vi "Main.vi"(8 "error in":errorcluster, 11 "gRPC Server in":refnum<class "gRPC Server.lvclass">) -> (0 "error out":errorcluster, 3 "gRPC Server out":refnum<class "gRPC Server.lvclass">)   [LabVIEW 2019, in "gRPC Server (template.proto).lvlib" / "gRPC Server.lvclass"]
doc: "The <b>Queued Message Handler</b> of the Worker that owns this VI."
uses:
  gRPC Server.lvclass
  C:/Program Files (x86)/National Instruments/LabVIEW 2019/vi.lib/addons/_Workers/Library/Classes/Worker/Worker.lvclass
  Generated_server/RPC Service/Session/Session.lvclass
  Generated_server/RPC Service/Session/Session.lvclass/Session.ctl
  rql_New Client Connection.ctl
  <vilib>/gRPC/LabVIEW gRPC Library/Shared/grpcId.ctl
  Initialization Data.ctl
  Response Cases.ctl
  <vilib>/addons/_Workers/Library/Case Label.ctl
  gRPC Server.lvclass/gRPC Server.ctl
  rsp_Connection Notify.ctl
  gRPC Read/Initialization Data.ctl
  gRPC Read/Response Cases.ctl
  rwr_Create gRPC Server.ctl
  rwr_Create gRPC Server Reply.ctl
  rwr_Destroy gRPC Server.ctl
  rwr_Destroy gRPC Server Reply.ctl
  rqp_Msg_ToClient_1.ctl
  Generated_server/RPC Messages/w4lvgrpc_Msg_ToClient_1.ctl
  Generated_server/RPC Messages/w4lvgrpc_ToClient.ctl
  Generated_server/RPC Messages/w4lvgrpc_ToClient_payload/w4lvgrpc_ToClient_payload.lvclass
  Generated_server/RPC Messages/w4lvgrpc_ToClient_payload/w4lvgrpc_ToClient_payload.lvclass/w4lvgrpc_ToClient_payload.ctl
  rqp_Msg_ToClient_2.ctl
  Generated_server/RPC Messages/w4lvgrpc_Msg_ToClient_2.ctl
  rqp_Msg_ToClient_3.ctl
  Generated_server/RPC Messages/w4lvgrpc_Msg_ToClient_3.ctl
  rqp_Msg_ToClient_4.ctl
  Generated_server/RPC Messages/w4lvgrpc_Msg_ToClient_4.ctl
  rqp_Msg_ToClient_5.ctl
  Generated_server/RPC Messages/w4lvgrpc_Msg_ToClient_5.ctl
  rqp_Msg_ToClient_6.ctl
  Generated_server/RPC Messages/w4lvgrpc_Msg_ToClient_6.ctl
  rqp_Msg_ToClient_7.ctl
  Generated_server/RPC Messages/w4lvgrpc_Msg_ToClient_7.ctl
  rqp_Msg_ToClient_8.ctl
  Generated_server/RPC Messages/w4lvgrpc_Msg_ToClient_8.ctl
  rqp_Msg_ToClient_9.ctl
  Generated_server/RPC Messages/w4lvgrpc_Msg_ToClient_9.ctl
  Generated_server/RPC Messages/w4lvgrpc_ToServer_payload/w4lvgrpc_ToServer_payload.lvclass/w4lvgrpc_ToServer_payload.ctl
  rsp_Msg_ToServer_1.ctl
  Generated_server/RPC Messages/w4lvgrpc_Msg_ToServer_1.ctl
  rsp_Msg_ToServer_2.ctl
  Generated_server/RPC Messages/w4lvgrpc_Msg_ToServer_2.ctl
  rsp_Msg_ToServer_3.ctl
  Generated_server/RPC Messages/w4lvgrpc_Msg_ToServer_3.ctl
  rsp_Msg_ToServer_4.ctl
  Generated_server/RPC Messages/w4lvgrpc_Msg_ToServer_4.ctl
  rsp_Msg_ToServer_5.ctl
  Generated_server/RPC Messages/w4lvgrpc_Msg_ToServer_5.ctl
  rsp_Msg_ToServer_6.ctl
  Generated_server/RPC Messages/w4lvgrpc_Msg_ToServer_6.ctl
  rsp_Msg_ToServer_7.ctl
  Generated_server/RPC Messages/w4lvgrpc_Msg_ToServer_7.ctl
  rsp_Msg_ToServer_8.ctl
  Generated_server/RPC Messages/w4lvgrpc_Msg_ToServer_8.ctl
  rsp_Msg_ToServer_9.ctl
  Generated_server/RPC Messages/w4lvgrpc_Msg_ToServer_9.ctl
  Generated_server/RPC Messages/Set w4lvgrpc_ToClient.vi
  Generated_server/RPC Messages/Set w4lvgrpc_ToClient.vi/dcc74a39-081a-4bdd-860b-8ed792803c96.vi
  Generated_server/RPC Messages/RichToFlatw4lvgrpc_ToClient.vi
  <vilib>/gRPC/LabVIEW gRPC Library/Shared/TranslateGrpcError.vi
  Generated_server/RPC Messages/RichToFlatw4lvgrpc_Msg_ToClient_1.vi
  Generated_server/RPC Messages/RichToFlatw4lvgrpc_Msg_ToClient_2.vi
  Generated_server/RPC Messages/RichToFlatw4lvgrpc_Msg_ToClient_3.vi
  Generated_server/RPC Messages/RichToFlatw4lvgrpc_Msg_ToClient_4.vi
  Generated_server/RPC Messages/RichToFlatw4lvgrpc_Msg_ToClient_5.vi
  Generated_server/RPC Messages/RichToFlatw4lvgrpc_Msg_ToClient_6.vi
  Generated_server/RPC Messages/RichToFlatw4lvgrpc_Msg_ToClient_7.vi
  Generated_server/RPC Messages/RichToFlatw4lvgrpc_Msg_ToClient_8.vi
  Generated_server/RPC Messages/RichToFlatw4lvgrpc_Msg_ToClient_9.vi
  <vilib>/Utility/error.llb/Error Cluster From Error Code.vi
  <vilib>/gRPC/LabVIEW gRPC Library/Server API/Server/Get Server DLL Path.vi
  <vilib>/addons/_Workers/Library/Classes/Message Queue/Message Queue.lvclass
  <vilib>/ErrorRing/Error Ring.xnode
  <vilib>/addons/_Workers/Library/Workers.lvlib
  gRPC Read/gRPC Read.lvclass
  Generated_server/RPC Messages/w4lvgrpc_ToServer_payload/w4lvgrpc_ToServer_payload.lvclass
  Generated_server/Generated_server.lvlib
  <vilib>/gRPC/LabVIEW gRPC Library/grpc-lvsupport-release.lvlib
  <vilib>/gRPC/LabVIEW gRPC Servicer/Servicer/Servicer.lvclass
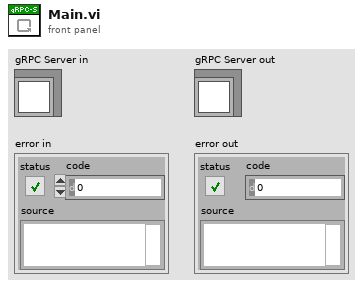
[diagram p1: front panel]
types:
  T1 = typedef "gRPC Server (template.proto).lvlib/gRPC Server.lvclass/rql_New Client Connection.ctl" = cluster{"gRPC ID":T2}
  T2 = typedef "grpc-lvsupport-release.lvlib/grpcId.ctl" = u64
  T3 = typedef "gRPC Server (template.proto).lvlib/gRPC Server.lvclass/Initialization Data.ctl" = cluster{"Response Cases":T4}
  T4 = typedef "gRPC Server (template.proto).lvlib/gRPC Server.lvclass/Response Cases.ctl" = cluster{"Connection Notify":T5, "Server Error":T5, "Msg_ToServer_1":T5, "Msg_ToServer_2":T5, "Msg_ToServer_3":T5, "Msg_ToServer_4":T5, "Msg_ToServer_5":T5, "Msg_ToServer_6":T5, "Msg_ToServer_7":T5, "Msg_ToServer_8":T5, "Msg_ToServer_9":T5}
  T5 = typedef "Workers.lvlib/Case Label.ctl" = string
  T6 = typedef "gRPC Server (template.proto).lvlib/gRPC Read.lvclass/Initialization Data.ctl" = cluster{"Response Cases":T7, "gRPC ID":T2}
  T7 = typedef "gRPC Server (template.proto).lvlib/gRPC Read.lvclass/Response Cases.ctl" = cluster{"Receive Incoming Data":T5, "Connection Lost":T5, "New Connection":T5}
  T8 = typedef "gRPC Server (template.proto).lvlib/gRPC Server.lvclass/rsp_Connection Notify.ctl" = cluster{"gRPC ID":T2, "Connected?":bool}
  T9 = typedef "gRPC Server (template.proto).lvlib/gRPC Server.lvclass/rwr_Create gRPC Server Reply.ctl" = cluster{"Listening Port":i32}
  T10 = typedef "gRPC Server (template.proto).lvlib/gRPC Server.lvclass/rwr_Create gRPC Server.ctl" = cluster{"Server Key File (.key)":path, "Server Certificate File (.crt)":path, "Server Address":string}
  T11 = typedef "gRPC Server (template.proto).lvlib/gRPC Server.lvclass/rwr_Destroy gRPC Server Reply.ctl" = cluster{"String":string}
  T12 = typedef "gRPC Server (template.proto).lvlib/gRPC Server.lvclass/rwr_Destroy gRPC Server.ctl" = cluster{"Placeholder":string}
  T13 = typedef "Generated_server.lvlib/w4lvgrpc_ToClient.ctl" = cluster{"w4lvgrpc_ToClient_payload":refnum<class "w4lvgrpc_ToClient_payload.lvclass">}
  T14 = typedef "gRPC Server (template.proto).lvlib/gRPC Server.lvclass/rqp_Msg_ToClient_1.ctl" = cluster{"w4lvgrpc_Msg_ToClient_1":T15}
  T15 = typedef "Generated_server.lvlib/w4lvgrpc_Msg_ToClient_1.ctl" = cluster{"placeholder":string}
  T16 = typedef "gRPC Server (template.proto).lvlib/gRPC Server.lvclass/rqp_Msg_ToClient_2.ctl" = cluster{"w4lvgrpc_Msg_ToClient_2":T17}
  T17 = typedef "Generated_server.lvlib/w4lvgrpc_Msg_ToClient_2.ctl" = cluster{"placeholder":string}
  T18 = typedef "gRPC Server (template.proto).lvlib/gRPC Server.lvclass/rqp_Msg_ToClient_3.ctl" = cluster{"w4lvgrpc_Msg_ToClient_3":T19}
  T19 = typedef "Generated_server.lvlib/w4lvgrpc_Msg_ToClient_3.ctl" = cluster{"placeholder":string}
  T20 = typedef "gRPC Server (template.proto).lvlib/gRPC Server.lvclass/rqp_Msg_ToClient_4.ctl" = cluster{"w4lvgrpc_Msg_ToClient_4":T21}
  T21 = typedef "Generated_server.lvlib/w4lvgrpc_Msg_ToClient_4.ctl" = cluster{"placeholder":string}
  T22 = typedef "gRPC Server (template.proto).lvlib/gRPC Server.lvclass/rqp_Msg_ToClient_5.ctl" = cluster{"w4lvgrpc_Msg_ToClient_5":T23}
  T23 = typedef "Generated_server.lvlib/w4lvgrpc_Msg_ToClient_5.ctl" = cluster{"placeholder":string}
  T24 = typedef "gRPC Server (template.proto).lvlib/gRPC Server.lvclass/rqp_Msg_ToClient_6.ctl" = cluster{"w4lvgrpc_Msg_ToClient_6":T25}
  T25 = typedef "Generated_server.lvlib/w4lvgrpc_Msg_ToClient_6.ctl" = cluster{"placeholder":string}
  T26 = typedef "gRPC Server (template.proto).lvlib/gRPC Server.lvclass/rqp_Msg_ToClient_7.ctl" = cluster{"w4lvgrpc_Msg_ToClient_7":T27}
  T27 = typedef "Generated_server.lvlib/w4lvgrpc_Msg_ToClient_7.ctl" = cluster{"placeholder":string}
  T28 = typedef "gRPC Server (template.proto).lvlib/gRPC Server.lvclass/rqp_Msg_ToClient_8.ctl" = cluster{"w4lvgrpc_Msg_ToClient_8":T29}
  T29 = typedef "Generated_server.lvlib/w4lvgrpc_Msg_ToClient_8.ctl" = cluster{"placeholder":string}
  T30 = typedef "gRPC Server (template.proto).lvlib/gRPC Server.lvclass/rqp_Msg_ToClient_9.ctl" = cluster{"w4lvgrpc_Msg_ToClient_9":T31}
  T31 = typedef "Generated_server.lvlib/w4lvgrpc_Msg_ToClient_9.ctl" = cluster{"placeholder":string}
  T32 = typedef "gRPC Server (template.proto).lvlib/gRPC Server.lvclass/rsp_Msg_ToServer_1.ctl" = cluster{"w4lvgrpc_Msg_ToServer_1":T33}
  T33 = typedef "Generated_server.lvlib/w4lvgrpc_Msg_ToServer_1.ctl" = cluster{"placeholder":string}
  T34 = typedef "gRPC Server (template.proto).lvlib/gRPC Server.lvclass/rsp_Msg_ToServer_2.ctl" = cluster{"w4lvgrpc_Msg_ToServer_2":T35}
  T35 = typedef "Generated_server.lvlib/w4lvgrpc_Msg_ToServer_2.ctl" = cluster{"placeholder":string}
  T36 = typedef "gRPC Server (template.proto).lvlib/gRPC Server.lvclass/rsp_Msg_ToServer_3.ctl" = cluster{"w4lvgrpc_Msg_ToServer_3":T37}
  T37 = typedef "Generated_server.lvlib/w4lvgrpc_Msg_ToServer_3.ctl" = cluster{"placeholder":string}
  T38 = typedef "gRPC Server (template.proto).lvlib/gRPC Server.lvclass/rsp_Msg_ToServer_4.ctl" = cluster{"w4lvgrpc_Msg_ToServer_4":T39}
  T39 = typedef "Generated_server.lvlib/w4lvgrpc_Msg_ToServer_4.ctl" = cluster{"placeholder":string}
  T40 = typedef "gRPC Server (template.proto).lvlib/gRPC Server.lvclass/rsp_Msg_ToServer_5.ctl" = cluster{"w4lvgrpc_Msg_ToServer_5":T41}
  T41 = typedef "Generated_server.lvlib/w4lvgrpc_Msg_ToServer_5.ctl" = cluster{"placeholder":string}
  T42 = typedef "gRPC Server (template.proto).lvlib/gRPC Server.lvclass/rsp_Msg_ToServer_6.ctl" = cluster{"w4lvgrpc_Msg_ToServer_6":T43}
  T43 = typedef "Generated_server.lvlib/w4lvgrpc_Msg_ToServer_6.ctl" = cluster{"placeholder":string}
  T44 = typedef "gRPC Server (template.proto).lvlib/gRPC Server.lvclass/rsp_Msg_ToServer_7.ctl" = cluster{"w4lvgrpc_Msg_ToServer_7":T45}
  T45 = typedef "Generated_server.lvlib/w4lvgrpc_Msg_ToServer_7.ctl" = cluster{"placeholder":string}
  T46 = typedef "gRPC Server (template.proto).lvlib/gRPC Server.lvclass/rsp_Msg_ToServer_8.ctl" = cluster{"w4lvgrpc_Msg_ToServer_8":T47}
  T47 = typedef "Generated_server.lvlib/w4lvgrpc_Msg_ToServer_8.ctl" = cluster{"placeholder":string}
  T48 = typedef "gRPC Server (template.proto).lvlib/gRPC Server.lvclass/rsp_Msg_ToServer_9.ctl" = cluster{"w4lvgrpc_Msg_ToServer_9":T49}
  T49 = typedef "Generated_server.lvlib/w4lvgrpc_Msg_ToServer_9.ctl" = cluster{"placeholder":string}
  T50 = typedef "gRPC Server (template.proto).lvlib/gRPC Read.lvclass/rsp_Receive Incoming Data.ctl" = refnum<class "w4lvgrpc_ToServer_payload.lvclass">
  T51 = typedef "Generated_server.lvlib/Session.lvclass/Server gRPC UEs.ctl" = cluster{"Session Connect gRPC UE":refnum<user-event>}
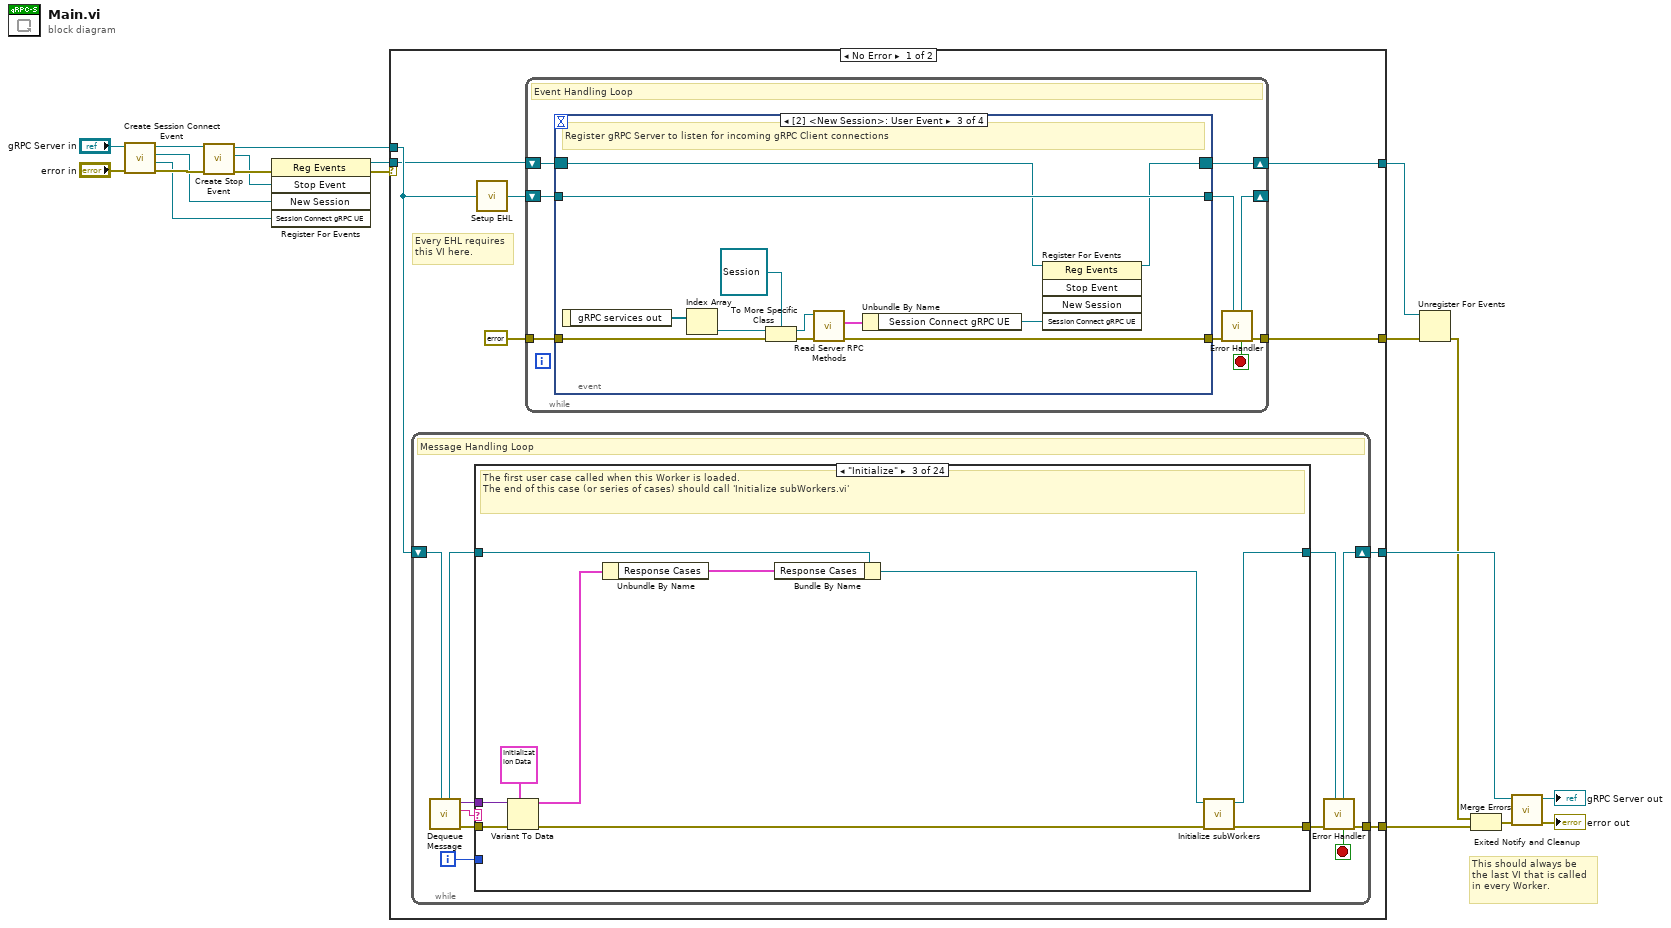
[diagram p0: block diagram]
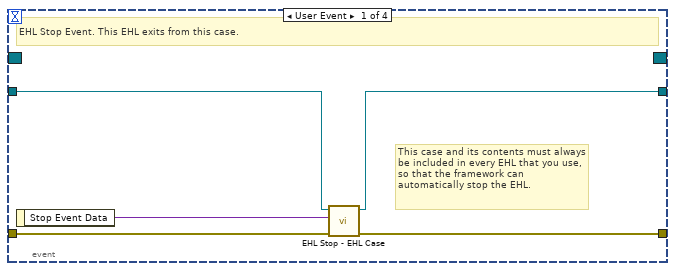
[diagram p2: hidden frame]
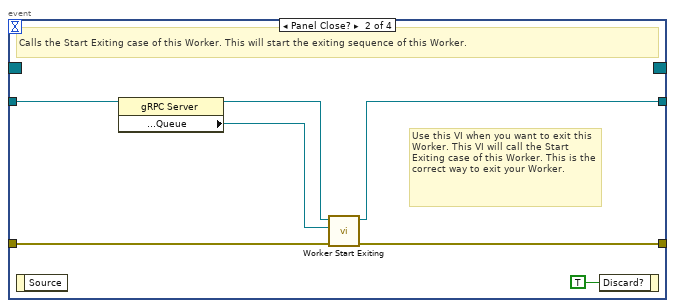
[diagram p3: hidden frame]
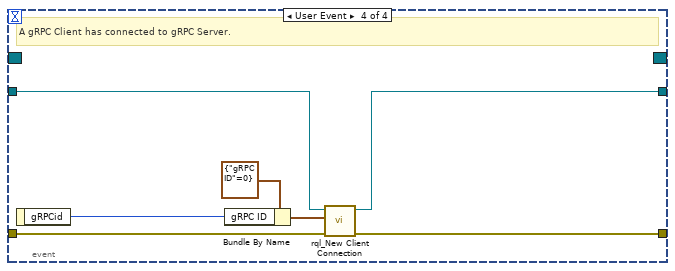
[diagram p4: hidden frame]
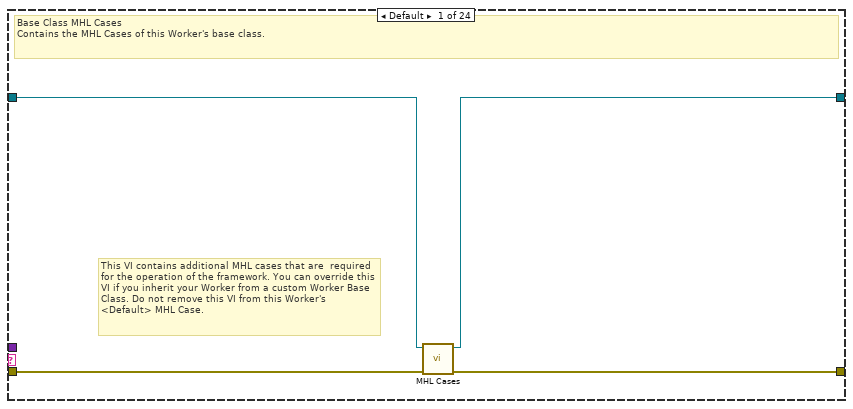
[diagram p5: hidden frame]
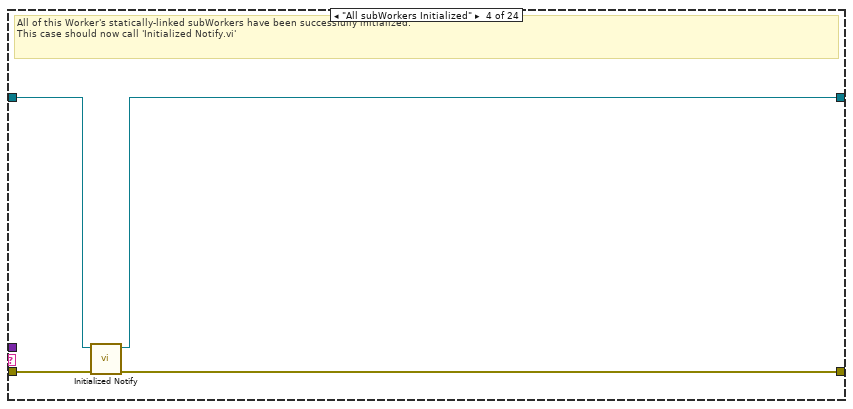
[diagram p7: hidden frame]
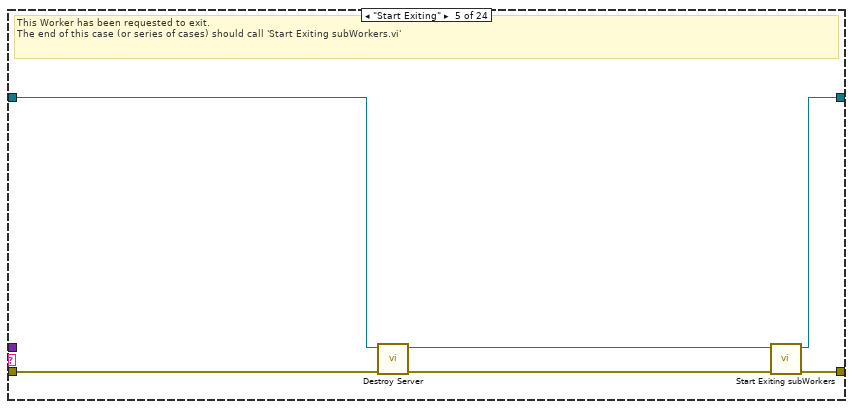
[diagram p8: hidden frame]
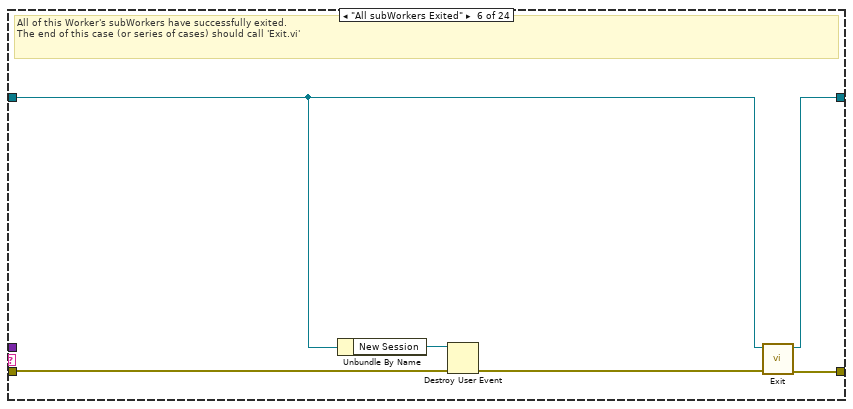
[diagram p9: hidden frame]
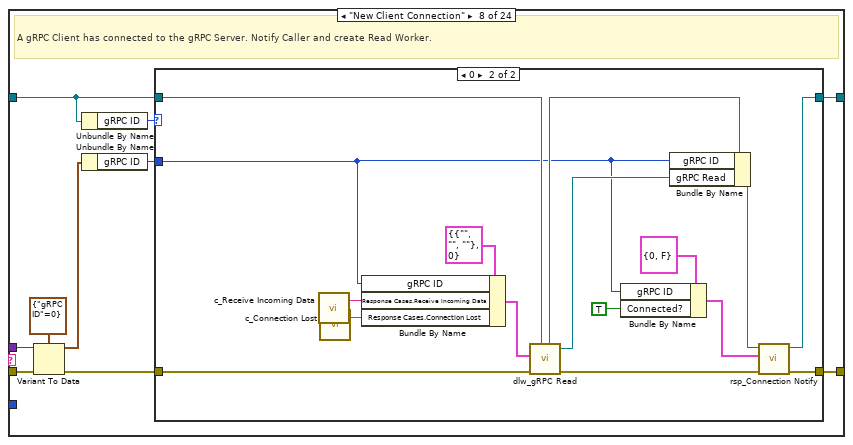
[diagram p11: hidden frame]
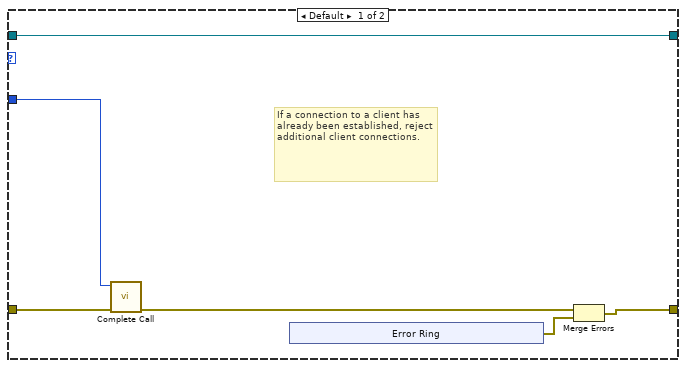
[diagram p12: hidden frame]
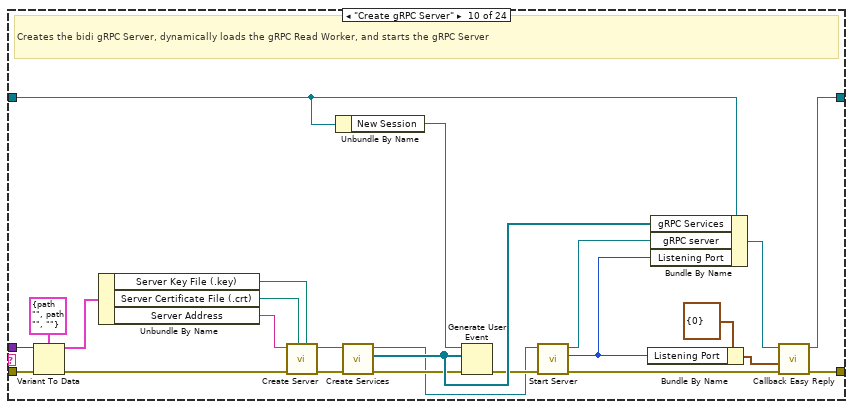
[diagram p14: hidden frame]
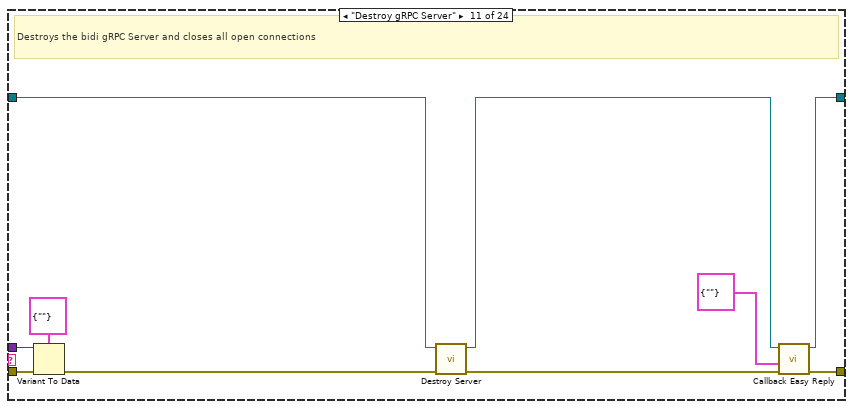
[diagram p15: hidden frame]
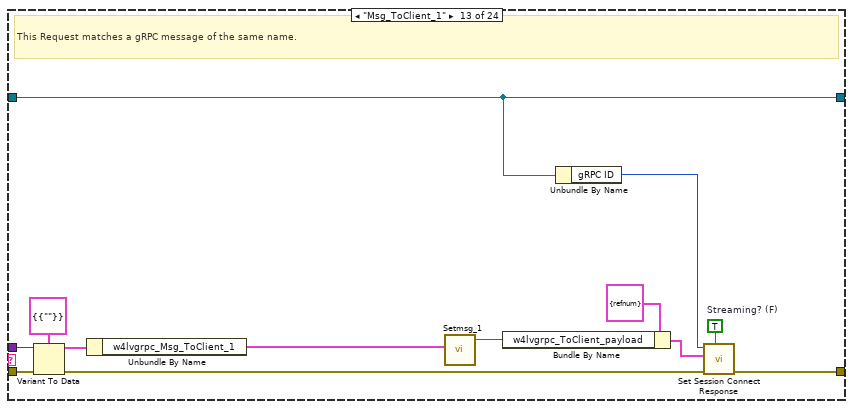
[diagram p17: hidden frame]
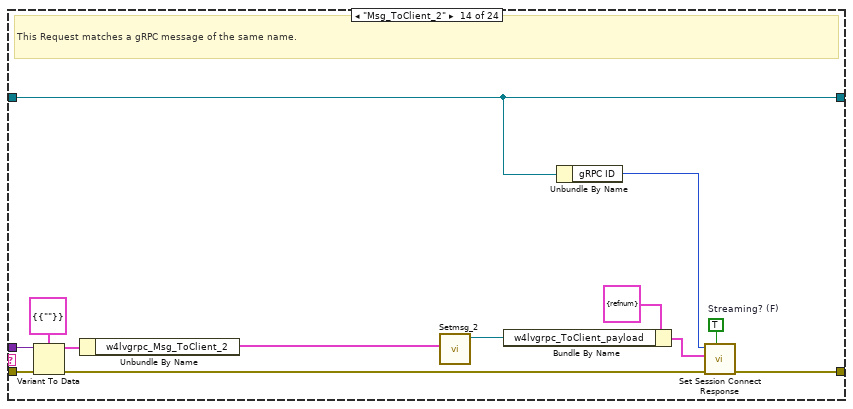
[diagram p18: hidden frame]
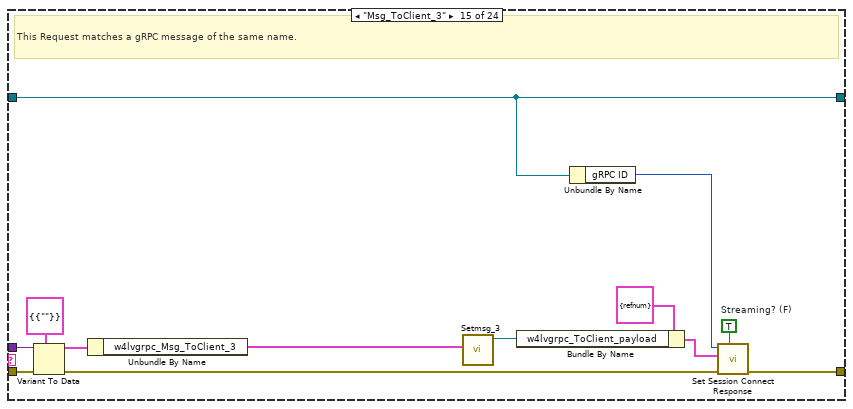
[diagram p19: hidden frame]
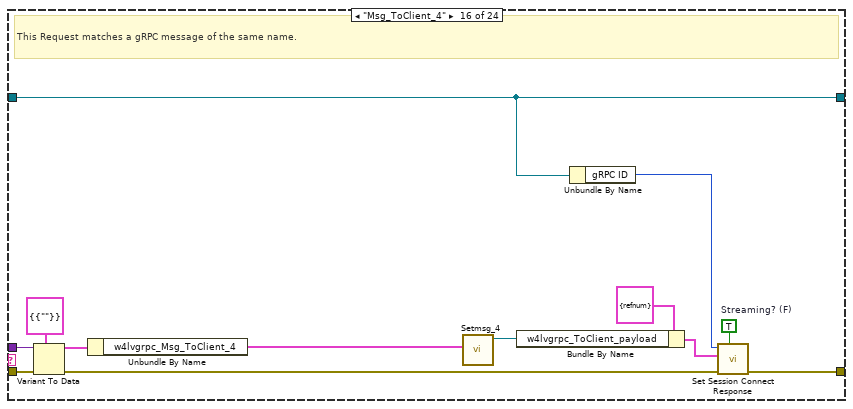
[diagram p20: hidden frame]
diagram:
  # "This should always be the last VI that is called in every Worker."
  n1 = call "Create Session Connect Event.vi"("error in (no error)"="error in", "gRPC Server in"="gRPC Server in") -> ("error out"=w4:errorcluster, "Session Connect gRPC UE"=w1:refnum<user-event>, "New Session"=w3:refnum<user-event>, "gRPC Server out"=w6:refnum<class "gRPC Server.lvclass">)  [unwired: 6 in]
  n2 = call-dynamic "Create Stop Event.vi"("error in"=w4, "Worker"=w6) -> ("error out"=w13:errorcluster, "Stop Event"=w5:refnum<user-event>, "Worker out"=w2:refnum<class "gRPC Server.lvclass">)  [unwired: 7 in]
  n3 = register-events(error in=w13, w5, w3, w1) -> (reference out=w12:refnum<event-registration>, error out=w14:errorcluster)  [unwired: 1 in]
  n4 = case shown="No Error" w14 {
    tunnel: w2 -> [w27 w426]
    tunnel: [w25 w427] -> w17
    tunnel: [w26 w425] -> w18
    selector: w14 -> [_ w428]
    tunnel: w12 -> [w22 w424]
    tunnel: [w21 w424] -> w11
    tunnel: [w20 w428] -> w10
    frame No Error {
      # "Every EHL requires\nthis VI here."
      n5 = while {
        shift-right: [w76] -> w26
        shift-left: w27 -> [w78]
        tunnel: [w77] -> w25
        i -> [w69]
        stop <- w70 stop-if-true
        # "Message Handling Loop"
        n6 = call-dynamic "Dequeue Message.vi"("Worker"=w78) -> ("error out"=w75:errorcluster, "Case out"=w71:string, "Data out"=w68:variant, "Worker out"=w73:refnum<class "gRPC Server.lvclass">)  [unwired: 6 in, 1 out]
        n7 = case "Worker MHL Case Structure (DO NOT CHANGE LABEL NAME)" shown="\"Initialize\"" w71 {
          tunnel: w75 -> [w82 w83 w92 w96 w102 w108 w112 w122 w151 w175 w185 w187 w200 w213 w226 w239 w252 w265 w278 w291 w304 w306 w312 w422]
          tunnel: [w81 w83 w94 w95 w104 w110 w112 w117 w151 w172 w182 w187 w191 w201 w220 w233 w246 w259 w272 w285 w298 w306 w316 w412] -> w74
          tunnel: w73 -> [w80 w84 w91 w98 w99 w107 w111 w115 w150 w157 w178 w186 w190 w205 w222 w235 w248 w261 w274 w287 w300 w305 w315 w421]
          tunnel: [w79 w84 w93 w97 w103 w109 w111 w118 w150 w171 w181 w186 w190 w205 w222 w235 w248 w261 w274 w287 w300 w305 w314 w410] -> w72
          tunnel: w69 -> [_ _ _ _ _ _ _ _ _ _ _ _ _ _ _ _ _ _ _ _ _ _ _ _]
          tunnel: w68 -> [_ _ w89 _ _ _ _ w120 _ w173 w183 _ w198 w211 w224 w237 w250 w263 w276 w289 w302 _ w313 w423]
          frame Default {
            # "This VI contains additional MHL cases that are  required for the operation of the framework. You can override this VI if you inherit your Worker from a custom Worker Base Class. Do not remove this VI from this Worker's <Default> MHL Case."
            # "Base Class MHL Cases\nContains the MHL Cases of this Worker's base class."
            n8 = call-dynamic "MHL Cases.vi"("error in"=w82, "Worker in"=w80) -> ("error out"=w81:errorcluster, "Worker out"=w79:refnum<class "gRPC Server.lvclass">)  [unwired: 8 in]
          }
          frame "------------ FRAMEWORK CASES -----------" {
            # "Start of Workers Framework Cases"
          }
          frame "Initialize" {
            # "The first user case called when this Worker is loaded.\nThe end of this case (or series of cases) should call 'Initialize subWorkers.vi'"
            n9 = Variant To Data(error in=w92, type=T3 {"Response Cases"={"Connection Notify"="", "Server Error"="", "Msg_ToServer_1"="", "Msg_ToServer_2"="", "Msg_ToServer_3"="", "Msg_ToServer_4"="", "Msg_ToServer_5"="", "Msg_ToServer_6"="", "Msg_ToServer_7"="", "Msg_ToServer_8"="", "Msg_ToServer_9"=""}} ("Initialization Data"), Variant=w89) -> (data=w88:T3, error out=w90:errorcluster)
            n10 = Unbundle By Name(w88) -> ("Response Cases"=w87:T4)
            n11 = Bundle By Name(cluster=w91, "Response Cases"=w87) -> (w85:refnum<class "gRPC Server.lvclass">)
            n12 = call-dynamic "Initialize subWorkers.vi"("error in"=w90, "Worker"=w85) -> ("error out"=w94:errorcluster, "dup Worker out"=w93:refnum<class "gRPC Server.lvclass">)  [unwired: 8 in]
          }
          frame "All subWorkers Initialized" {
            # "All of this Worker's statically-linked subWorkers have been successfully initialized.\nThis case should now call 'Initialized Notify.vi'"
            n13 = call-dynamic "Initialized Notify.vi"("error in"=w96, "Worker"=w98) -> ("error out"=w95:errorcluster, "dup Worker out"=w97:refnum<class "gRPC Server.lvclass">)  [unwired: 8 in]
          }
          frame "Start Exiting" {
            # "This Worker has been requested to exit. \nThe end of this case (or series of cases) should call 'Start Exiting subWorkers.vi'"
            n14 = call "Destroy Server.vi"("error in (no error)"=w102, "gRPC Server in"=w99) -> ("error out"=w101:errorcluster, "gRPC Server out"=w100:refnum<class "gRPC Server.lvclass">)  [unwired: 8 in]
            n15 = call-dynamic "Start Exiting subWorkers.vi"("error_in"=w101, "Worker"=w100) -> ("error out"=w104:errorcluster, "dup Worker out"=w103:refnum<class "gRPC Server.lvclass">)  [unwired: 8 in]
          }
          frame "All subWorkers Exited" {
            # "All of this Worker's subWorkers have successfully exited. \nThe end of this case (or series of cases) should call 'Exit.vi'"
            n16 = Unbundle By Name(w107) -> ("New Session"=w106:refnum<user-event>)
            n17 = Destroy User Event(user event=w106, error in=w108) -> (error out=w105:errorcluster)
            n18 = call-dynamic "Exit.vi"("error_in"=w105, "Worker"=w107) -> ("error out"=w110:errorcluster, "dup Worker out"=w109:refnum<class "gRPC Server.lvclass">)  [unwired: 8 in]
          }
          frame "------------- LOCAL API CASES -------------" {
            # "Start of Workers Local API Cases"
          }
          frame "New Client Connection" {
            # "A gRPC Client has connected to the gRPC Server. Notify Caller and create Read Worker."
            n19 = Variant To Data(error in=w122, type=T1 {"gRPC ID"=0} ("Data"), Variant=w120) -> (data=w119:T1, error out=w116:errorcluster)
            n20 = Unbundle By Name(w115) -> ("gRPC ID"=w114:T2)
            n21 = Unbundle By Name(w119) -> ("gRPC ID"=w113:T2)
            n22 = case shown="0" w114 {
              tunnel: [w128 w145] -> w118
              tunnel: [w125 w144] -> w117
              tunnel: w115 -> [w128 w139]
              tunnel: w116 -> [w126 w138]
              tunnel: w113 -> [w123 w134]
              frame Default {
                # "If a connection to a client has already been established, reject additional client connections."
                n23 = call <vilib>:"Complete Call.vi"("gRPCid"=w123, "error in"=w126) -> ("error out"=w127:errorcluster)  [unwired: 8 in]
                n24 = xnode "Error Ring"() -> ("error out"=w124:errorcluster)
                n25 = Merge Errors(w127, w124) -> (w125:errorcluster)
              }
              frame 0 {
                n26 = call "c_Receive Incoming Data.vi"() -> ("Case Label"=w142:T5)  [unwired: 1 in]
                n27 = call "c_Connection Lost.vi"() -> ("Case Label"=w141:T5)  [unwired: 1 in]
                n28 = Bundle By Name(cluster=T6 {"Response Cases"={"Receive Incoming Data"="", "Connection Lost"="", "New Connection"=""}, "gRPC ID"=0} ("Initialization Data"), "gRPC ID"=w134, "Response Cases.Receive Incoming Data"=w142, "Response Cases.Connection Lost"=w141) -> (w137:T6)
                n29 = call "dlw_gRPC Read.vi"("Caller in"=w139, "error in"=w138, "Initialization Data"=w137) -> ("error out"=w136:errorcluster, "gRPC Read out"=w135:refnum<class "gRPC Read.lvclass">, "dup Caller out"=w140:refnum<class "gRPC Server.lvclass">)  [unwired: 6 in]
                n30 = Bundle By Name(cluster=T8 {"gRPC ID"=0, "Connected?"=FALSE} ("Data in"), "gRPC ID"=w134, "Connected?"=TRUE) -> (w148:T8)
                n31 = Bundle By Name(cluster=w140, "gRPC ID"=w134, "gRPC Read"=w135) -> (w146:refnum<class "gRPC Server.lvclass">)
                n32 = call "rsp_Connection Notify.vi"("error in"=w136, "Data in"=w148, "gRPC Server in"=w146) -> ("error out"=w144:errorcluster, "dup gRPC Server out"=w145:refnum<class "gRPC Server.lvclass">)  [unwired: 7 in]
              }
            }
          }
          frame "------------- PUBLIC API CASES -------------" {
            # "Start of Workers Public API Cases"
          }
          frame "Create gRPC Server" {
            # "Creates the bidi gRPC Server, dynamically loads the gRPC Read Worker, and starts the gRPC Server"
            n33 = Variant To Data(error in=w175, type=T10 {"Server Key File (.key)"=path "", "Server Certificate File (.crt)"=path "", "Server Address"=""} ("Data"), Variant=w173) -> (data=w155:T10, error out=w156:errorcluster)
            n34 = Unbundle By Name(w155) -> ("Server Key File (.key)"=w165:path, "Server Certificate File (.crt)"=w164:path, "Server Address"=w163:string)
            n35 = call <vilib>:"Create Server.vi"("Server Key File (.key)"=w165, "Server Certificate File (.crt)"=w164, "error in"=w156, "Server Address"=w163) -> ("error out"=w162:errorcluster, "gRPC server out"=w161:refnum<class "Servicer.lvclass">)  [unwired: 6 in]
            n36 = Unbundle By Name(w157) -> ("New Session"=w167:refnum<user-event>)
            n37 = call "Create Services.vi"("error in (no error)"=w162, "gRPC server in"=w161) -> ("error out"=w168:errorcluster, "gRPC services out"=w170:refnum<class "ServiceBase.lvclass">[], "gRPC server out"=w160:refnum<class "Servicer.lvclass">)  [unwired: 7 in]
            n38 = Generate User Event(user event=w167, event data cluster=w170, error in=w168) -> (error out=w169:errorcluster)  [unwired: 1 in, 1 out]
            n39 = call <vilib>:"Start Server.vi"("error in"=w169, "gRPC server in"=w160) -> ("error out"=w154:errorcluster, "Listening Port"=w159:i32, "gRPC server out"=w158:refnum<class "Servicer.lvclass">)  [unwired: 7 in]
            n40 = Bundle By Name(cluster=T9 {"Listening Port"=0} ("Reply Data"), "Listening Port"=w159) -> (w152:T9)
            n41 = Bundle By Name(cluster=w157, "gRPC Services"=w170, "gRPC server"=w158, "Listening Port"=w159) -> (w153:refnum<class "gRPC Server.lvclass">)
            n42 = call-dynamic "Callback Easy Reply.vi"("error in"=w154, "Data"=w152, "Worker"=w153) -> ("error out"=w172:errorcluster, "dup Worker out"=w171:refnum<class "gRPC Server.lvclass">)  [unwired: 7 in]
          }
          frame "Destroy gRPC Server" {
            # "Destroys the bidi gRPC Server and closes all open connections"
            n43 = Variant To Data(error in=w185, type=T12 {"Placeholder"=""} ("Data"), Variant=w183) -> (error out=w179:errorcluster)  [unwired: 1 out]
            n44 = call "Destroy Server.vi"("error in (no error)"=w179, "gRPC Server in"=w178) -> ("error out"=w177:errorcluster, "gRPC Server out"=w176:refnum<class "gRPC Server.lvclass">)  [unwired: 8 in]
            n45 = call-dynamic "Callback Easy Reply.vi"("error in"=w177, "Data"=T11 {"String"=""} ("Reply Data"), "Worker"=w176) -> ("error out"=w182:errorcluster, "dup Worker out"=w181:refnum<class "gRPC Server.lvclass">)  [unwired: 7 in]
          }
          frame "~~~~~~~~ gRPC Messages ~~~~~~~~~~ " {
          }
          frame "Msg_ToClient_1" {
            w195 = TRUE  # Streaming? (F)
            # "This Request matches a gRPC message of the same name."
            n46 = Variant To Data(error in=w200, type=T14 {"w4lvgrpc_Msg_ToClient_1"={"placeholder"=""}} ("Data"), Variant=w198) -> (data=w197:T14, error out=w192:errorcluster)
            n47 = Unbundle By Name(w197) -> ("w4lvgrpc_Msg_ToClient_1"=w188:T15)
            n48 = call "Setmsg_1.vi"("Set_Val"=w188) -> ("OneOfTemplate out"=w189:refnum<class "w4lvgrpc_ToClient_payload.lvclass">)  [unwired: 9 in, 1 out]
            n49 = Bundle By Name(cluster=T13 {"w4lvgrpc_ToClient_payload"=refnum} ("Message Data"), "w4lvgrpc_ToClient_payload"=w189) -> (w193:T13)
            n50 = Unbundle By Name(w190) -> ("gRPC ID"=w196:T2)
            n51 = call "Set Session Connect Response.vi"("Streaming? (F)"=w195, "error in (no error)"=w192, "Message Data"=w193, "gRPCid in"=w196) -> ("error out"=w191:errorcluster)  [unwired: 7 in]
          }
          frame "Msg_ToClient_2" {
            w208 = TRUE  # Streaming? (F)
            # "This Request matches a gRPC message of the same name."
            n52 = Variant To Data(error in=w213, type=T16 {"w4lvgrpc_Msg_ToClient_2"={"placeholder"=""}} ("Data"), Variant=w211) -> (data=w210:T16, error out=w202:errorcluster)
            n53 = Unbundle By Name(w210) -> ("w4lvgrpc_Msg_ToClient_2"=w203:T17)
            n54 = call "Setmsg_2.vi"("Set_Val"=w203) -> ("OneOfTemplate out"=w204:refnum<class "w4lvgrpc_ToClient_payload.lvclass">)  [unwired: 9 in, 1 out]
            n55 = Bundle By Name(cluster=T13 {"w4lvgrpc_ToClient_payload"=refnum} ("Message Data"), "w4lvgrpc_ToClient_payload"=w204) -> (w206:T13)
            n56 = Unbundle By Name(w205) -> ("gRPC ID"=w209:T2)
            n57 = call "Set Session Connect Response.vi"("Streaming? (F)"=w208, "error in (no error)"=w202, "Message Data"=w206, "gRPCid in"=w209) -> ("error out"=w201:errorcluster)  [unwired: 7 in]
          }
          frame "Msg_ToClient_3" {
            w218 = TRUE  # Streaming? (F)
            # "This Request matches a gRPC message of the same name."
            n58 = Variant To Data(error in=w226, type=T18 {"w4lvgrpc_Msg_ToClient_3"={"placeholder"=""}} ("Data"), Variant=w224) -> (data=w223:T18, error out=w219:errorcluster)
            n59 = Unbundle By Name(w223) -> ("w4lvgrpc_Msg_ToClient_3"=w215:T19)
            n60 = call "Setmsg_3.vi"("Set_Val"=w215) -> ("OneOfTemplate out"=w214:refnum<class "w4lvgrpc_ToClient_payload.lvclass">)  [unwired: 9 in, 1 out]
            n61 = Bundle By Name(cluster=T13 {"w4lvgrpc_ToClient_payload"=refnum} ("Message Data"), "w4lvgrpc_ToClient_payload"=w214) -> (w216:T13)
            n62 = Unbundle By Name(w222) -> ("gRPC ID"=w221:T2)
            n63 = call "Set Session Connect Response.vi"("Streaming? (F)"=w218, "error in (no error)"=w219, "Message Data"=w216, "gRPCid in"=w221) -> ("error out"=w220:errorcluster)  [unwired: 7 in]
          }
          frame "Msg_ToClient_4" {
            w231 = TRUE  # Streaming? (F)
            # "This Request matches a gRPC message of the same name."
            n64 = Variant To Data(error in=w239, type=T20 {"w4lvgrpc_Msg_ToClient_4"={"placeholder"=""}} ("Data"), Variant=w237) -> (data=w236:T20, error out=w232:errorcluster)
            n65 = Unbundle By Name(w236) -> ("w4lvgrpc_Msg_ToClient_4"=w227:T21)
            n66 = call "Setmsg_4.vi"("Set_Val"=w227) -> ("OneOfTemplate out"=w228:refnum<class "w4lvgrpc_ToClient_payload.lvclass">)  [unwired: 9 in, 1 out]
            n67 = Bundle By Name(cluster=T13 {"w4lvgrpc_ToClient_payload"=refnum} ("Message Data"), "w4lvgrpc_ToClient_payload"=w228) -> (w229:T13)
            n68 = Unbundle By Name(w235) -> ("gRPC ID"=w234:T2)
            n69 = call "Set Session Connect Response.vi"("Streaming? (F)"=w231, "error in (no error)"=w232, "Message Data"=w229, "gRPCid in"=w234) -> ("error out"=w233:errorcluster)  [unwired: 7 in]
          }
          frame "Msg_ToClient_5" {
            w244 = TRUE  # Streaming? (F)
            # "This Request matches a gRPC message of the same name."
            n70 = Variant To Data(error in=w252, type=T22 {"w4lvgrpc_Msg_ToClient_5"={"placeholder"=""}} ("Data"), Variant=w250) -> (data=w249:T22, error out=w245:errorcluster)
            n71 = Unbundle By Name(w249) -> ("w4lvgrpc_Msg_ToClient_5"=w240:T23)
            n72 = call "Setmsg_5.vi"("Set_Val"=w240) -> ("OneOfTemplate out"=w241:refnum<class "w4lvgrpc_ToClient_payload.lvclass">)  [unwired: 9 in, 1 out]
            n73 = Bundle By Name(cluster=T13 {"w4lvgrpc_ToClient_payload"=refnum} ("Message Data"), "w4lvgrpc_ToClient_payload"=w241) -> (w242:T13)
            n74 = Unbundle By Name(w248) -> ("gRPC ID"=w247:T2)
            n75 = call "Set Session Connect Response.vi"("Streaming? (F)"=w244, "error in (no error)"=w245, "Message Data"=w242, "gRPCid in"=w247) -> ("error out"=w246:errorcluster)  [unwired: 7 in]
          }
          frame "Msg_ToClient_6" {
            w257 = TRUE  # Streaming? (F)
            # "This Request matches a gRPC message of the same name."
            n76 = Variant To Data(error in=w265, type=T24 {"w4lvgrpc_Msg_ToClient_6"={"placeholder"=""}} ("Data"), Variant=w263) -> (data=w262:T24, error out=w258:errorcluster)
            n77 = Unbundle By Name(w262) -> ("w4lvgrpc_Msg_ToClient_6"=w253:T25)
            n78 = call "Setmsg_6.vi"("Set_Val"=w253) -> ("OneOfTemplate out"=w254:refnum<class "w4lvgrpc_ToClient_payload.lvclass">)  [unwired: 9 in, 1 out]
            n79 = Bundle By Name(cluster=T13 {"w4lvgrpc_ToClient_payload"=refnum} ("Message Data"), "w4lvgrpc_ToClient_payload"=w254) -> (w255:T13)
            n80 = Unbundle By Name(w261) -> ("gRPC ID"=w260:T2)
            n81 = call "Set Session Connect Response.vi"("Streaming? (F)"=w257, "error in (no error)"=w258, "Message Data"=w255, "gRPCid in"=w260) -> ("error out"=w259:errorcluster)  [unwired: 7 in]
          }
          frame "Msg_ToClient_7" {
            w270 = TRUE  # Streaming? (F)
            # "This Request matches a gRPC message of the same name."
            n82 = Variant To Data(error in=w278, type=T26 {"w4lvgrpc_Msg_ToClient_7"={"placeholder"=""}} ("Data"), Variant=w276) -> (data=w275:T26, error out=w271:errorcluster)
            n83 = Unbundle By Name(w275) -> ("w4lvgrpc_Msg_ToClient_7"=w266:T27)
            n84 = call "Setmsg_7.vi"("Set_Val"=w266) -> ("OneOfTemplate out"=w267:refnum<class "w4lvgrpc_ToClient_payload.lvclass">)  [unwired: 9 in, 1 out]
            n85 = Bundle By Name(cluster=T13 {"w4lvgrpc_ToClient_payload"=refnum} ("Message Data"), "w4lvgrpc_ToClient_payload"=w267) -> (w268:T13)
            n86 = Unbundle By Name(w274) -> ("gRPC ID"=w273:T2)
            n87 = call "Set Session Connect Response.vi"("Streaming? (F)"=w270, "error in (no error)"=w271, "Message Data"=w268, "gRPCid in"=w273) -> ("error out"=w272:errorcluster)  [unwired: 7 in]
          }
          frame "Msg_ToClient_8" {
            w283 = TRUE  # Streaming? (F)
            # "This Request matches a gRPC message of the same name."
            n88 = Variant To Data(error in=w291, type=T28 {"w4lvgrpc_Msg_ToClient_8"={"placeholder"=""}} ("Data"), Variant=w289) -> (data=w288:T28, error out=w284:errorcluster)
            n89 = Unbundle By Name(w288) -> ("w4lvgrpc_Msg_ToClient_8"=w279:T29)
            n90 = call "Setmsg_8.vi"("Set_Val"=w279) -> ("OneOfTemplate out"=w280:refnum<class "w4lvgrpc_ToClient_payload.lvclass">)  [unwired: 9 in, 1 out]
            n91 = Bundle By Name(cluster=T13 {"w4lvgrpc_ToClient_payload"=refnum} ("Message Data"), "w4lvgrpc_ToClient_payload"=w280) -> (w281:T13)
            n92 = Unbundle By Name(w287) -> ("gRPC ID"=w286:T2)
            n93 = call "Set Session Connect Response.vi"("Streaming? (F)"=w283, "error in (no error)"=w284, "Message Data"=w281, "gRPCid in"=w286) -> ("error out"=w285:errorcluster)  [unwired: 7 in]
          }
          frame "Msg_ToClient_9" {
            w296 = TRUE  # Streaming? (F)
            # "This Request matches a gRPC message of the same name."
            n94 = Variant To Data(error in=w304, type=T30 {"w4lvgrpc_Msg_ToClient_9"={"placeholder"=""}} ("Data"), Variant=w302) -> (data=w301:T30, error out=w297:errorcluster)
            n95 = Unbundle By Name(w301) -> ("w4lvgrpc_Msg_ToClient_9"=w292:T31)
            n96 = call "Setmsg_9.vi"("Set_Val"=w292) -> ("OneOfTemplate out"=w293:refnum<class "w4lvgrpc_ToClient_payload.lvclass">)  [unwired: 9 in, 1 out]
            n97 = Bundle By Name(cluster=T13 {"w4lvgrpc_ToClient_payload"=refnum} ("Message Data"), "w4lvgrpc_ToClient_payload"=w293) -> (w294:T13)
            n98 = Unbundle By Name(w300) -> ("gRPC ID"=w299:T2)
            n99 = call "Set Session Connect Response.vi"("Streaming? (F)"=w296, "error in (no error)"=w297, "Message Data"=w294, "gRPCid in"=w299) -> ("error out"=w298:errorcluster)  [unwired: 7 in]
          }
          frame "------------- RESPONSE CASES --------------" {
            # "Start of Workers Response Cases"
          }
          frame "Receive Incoming Data" {
            # "*** IMPORTANT ***\n\nCase Selector must match index of gRPC ProtoBuf ToServer oneof payload"
            # "This case receives incoming data from a gRPC Client, and then delegates the data to the associated Public Response"
            n100 = call "rspvtd_Receive Incoming Data.vi"("error in"=w312, "Data in"=w313) -> ("error out"=w310:errorcluster, "Data out"=w311:T50)  [unwired: 8 in]
            n101 = call "GetActiveFieldIndex.vi"("error in (no error)"=w310, "OneOfTemplate in"=w311) -> ("error out"=w307:errorcluster, "Active Field Index"=w308:i32, "OneOfTemplate out"=w309:T50)  [unwired: 7 in]
            n102 = case shown="1" w308 {
              selector: w308 -> [w317 _ _ _ _ _ _ _ _ _]
              tunnel: w307 -> [w318 w333 w342 w351 w360 w369 w378 w387 w396 w405]
              tunnel: [w319 w337 w346 w355 w364 w373 w382 w391 w400 w409] -> w316
              tunnel: w315 -> [w321 w336 w345 w354 w363 w372 w381 w390 w399 w408]
              tunnel: [w321 w335 w344 w353 w362 w371 w380 w389 w398 w407] -> w314
              tunnel: w309 -> [_ w334 w343 w352 w361 w370 w379 w388 w397 w406]
              frame Default {
                n103 = xnode "Error Ring"("parameter 0"=w317) -> ("error out"=w320:errorcluster)
                n104 = Merge Errors(w318, w320) -> (w319:errorcluster)
              }
              frame 1 {
                n105 = call "Getmsg_1.vi"("error in (no error)"=w333, "OneOfTemplate in"=w334) -> ("error out"=w332:errorcluster, "Get_Val"=w329:T33)  [unwired: 7 in, 1 out]
                n106 = Bundle By Name(cluster=T32 {"w4lvgrpc_Msg_ToServer_1"={"placeholder"=""}} ("Data in"), "w4lvgrpc_Msg_ToServer_1"=w329) -> (w330:T32)
                n107 = call "rsp_Msg_ToServer_1.vi"("error in"=w332, "Data in"=w330, "gRPC Server in"=w336) -> ("error out"=w337:errorcluster, "dup gRPC Server out"=w335:refnum<class "gRPC Server.lvclass">)  [unwired: 7 in]
              }
              frame 2 {
                n108 = call "Getmsg_2.vi"("error in (no error)"=w342, "OneOfTemplate in"=w343) -> ("error out"=w341:errorcluster, "Get_Val"=w338:T35)  [unwired: 7 in, 1 out]
                n109 = Bundle By Name(cluster=T34 {"w4lvgrpc_Msg_ToServer_2"={"placeholder"=""}} ("Data in"), "w4lvgrpc_Msg_ToServer_2"=w338) -> (w339:T34)
                n110 = call "rsp_Msg_ToServer_2.vi"("error in"=w341, "Data in"=w339, "gRPC Server in"=w345) -> ("error out"=w346:errorcluster, "dup gRPC Server out"=w344:refnum<class "gRPC Server.lvclass">)  [unwired: 7 in]
              }
              frame 3 {
                n111 = call "Getmsg_3.vi"("error in (no error)"=w351, "OneOfTemplate in"=w352) -> ("error out"=w350:errorcluster, "Get_Val"=w347:T37)  [unwired: 7 in, 1 out]
                n112 = Bundle By Name(cluster=T36 {"w4lvgrpc_Msg_ToServer_3"={"placeholder"=""}} ("Data in"), "w4lvgrpc_Msg_ToServer_3"=w347) -> (w348:T36)
                n113 = call "rsp_Msg_ToServer_3.vi"("error in"=w350, "Data in"=w348, "gRPC Server in"=w354) -> ("error out"=w355:errorcluster, "dup gRPC Server out"=w353:refnum<class "gRPC Server.lvclass">)  [unwired: 7 in]
              }
              frame 4 {
                n114 = call "Getmsg_4.vi"("error in (no error)"=w360, "OneOfTemplate in"=w361) -> ("error out"=w359:errorcluster, "Get_Val"=w356:T39)  [unwired: 7 in, 1 out]
                n115 = Bundle By Name(cluster=T38 {"w4lvgrpc_Msg_ToServer_4"={"placeholder"=""}} ("Data in"), "w4lvgrpc_Msg_ToServer_4"=w356) -> (w357:T38)
                n116 = call "rsp_Msg_ToServer_4.vi"("error in"=w359, "Data in"=w357, "gRPC Server in"=w363) -> ("error out"=w364:errorcluster, "dup gRPC Server out"=w362:refnum<class "gRPC Server.lvclass">)  [unwired: 7 in]
              }
              frame 5 {
                n117 = call "Getmsg_5.vi"("error in (no error)"=w369, "OneOfTemplate in"=w370) -> ("error out"=w368:errorcluster, "Get_Val"=w365:T41)  [unwired: 7 in, 1 out]
                n118 = Bundle By Name(cluster=T40 {"w4lvgrpc_Msg_ToServer_5"={"placeholder"=""}} ("Data in"), "w4lvgrpc_Msg_ToServer_5"=w365) -> (w366:T40)
                n119 = call "rsp_Msg_ToServer_5.vi"("error in"=w368, "Data in"=w366, "gRPC Server in"=w372) -> ("error out"=w373:errorcluster, "dup gRPC Server out"=w371:refnum<class "gRPC Server.lvclass">)  [unwired: 7 in]
              }
              frame 6 {
                n120 = call "Getmsg_6.vi"("error in (no error)"=w378, "OneOfTemplate in"=w379) -> ("error out"=w377:errorcluster, "Get_Val"=w374:T43)  [unwired: 7 in, 1 out]
                n121 = Bundle By Name(cluster=T42 {"w4lvgrpc_Msg_ToServer_6"={"placeholder"=""}} ("Data in"), "w4lvgrpc_Msg_ToServer_6"=w374) -> (w375:T42)
                n122 = call "rsp_Msg_ToServer_6.vi"("error in"=w377, "Data in"=w375, "gRPC Server in"=w381) -> ("error out"=w382:errorcluster, "dup gRPC Server out"=w380:refnum<class "gRPC Server.lvclass">)  [unwired: 7 in]
              }
              frame 7 {
                n123 = call "Getmsg_7.vi"("error in (no error)"=w387, "OneOfTemplate in"=w388) -> ("error out"=w386:errorcluster, "Get_Val"=w383:T45)  [unwired: 7 in, 1 out]
                n124 = Bundle By Name(cluster=T44 {"w4lvgrpc_Msg_ToServer_7"={"placeholder"=""}} ("Data in"), "w4lvgrpc_Msg_ToServer_7"=w383) -> (w384:T44)
                n125 = call "rsp_Msg_ToServer_7.vi"("error in"=w386, "Data in"=w384, "gRPC Server in"=w390) -> ("error out"=w391:errorcluster, "dup gRPC Server out"=w389:refnum<class "gRPC Server.lvclass">)  [unwired: 7 in]
              }
              frame 8 {
                n126 = call "Getmsg_8.vi"("error in (no error)"=w396, "OneOfTemplate in"=w397) -> ("error out"=w395:errorcluster, "Get_Val"=w392:T47)  [unwired: 7 in, 1 out]
                n127 = Bundle By Name(cluster=T46 {"w4lvgrpc_Msg_ToServer_8"={"placeholder"=""}} ("Data in"), "w4lvgrpc_Msg_ToServer_8"=w392) -> (w393:T46)
                n128 = call "rsp_Msg_ToServer_8.vi"("error in"=w395, "Data in"=w393, "gRPC Server in"=w399) -> ("error out"=w400:errorcluster, "dup gRPC Server out"=w398:refnum<class "gRPC Server.lvclass">)  [unwired: 7 in]
              }
              frame 9 {
                n129 = call "Getmsg_9.vi"("error in (no error)"=w405, "OneOfTemplate in"=w406) -> ("error out"=w404:errorcluster, "Get_Val"=w401:T49)  [unwired: 7 in, 1 out]
                n130 = Bundle By Name(cluster=T48 {"w4lvgrpc_Msg_ToServer_9"={"placeholder"=""}} ("Data in"), "w4lvgrpc_Msg_ToServer_9"=w401) -> (w402:T48)
                n131 = call "rsp_Msg_ToServer_9.vi"("error in"=w404, "Data in"=w402, "gRPC Server in"=w408) -> ("error out"=w409:errorcluster, "dup gRPC Server out"=w407:refnum<class "gRPC Server.lvclass">)  [unwired: 7 in]
              }
            }
          }
          frame "Connection Lost" {
            w415 = T2 0 ("gRPC ID")
            # "A connection to the gRPC Client has been lost. Notify Caller and exit Read Worker."
            n132 = call "rspvtd_Connection Lost.vi"("error in"=w422, "Data in"=w423) -> ("error out"=w416:errorcluster)  [unwired: 8 in, 1 out]
            n133 = Bundle By Name(cluster=T8 {"gRPC ID"=0, "Connected?"=FALSE} ("Data in"), "gRPC ID"=w415, "Connected?"=FALSE) -> (w418:T8)
            n134 = Bundle By Name(cluster=w421, "gRPC ID"=w415) -> (w420:refnum<class "gRPC Server.lvclass">)
            n135 = call "rsp_Connection Notify.vi"("error in"=w416, "Data in"=w418, "gRPC Server in"=w420) -> ("error out"=w413:errorcluster, "dup gRPC Server out"=w411:refnum<class "gRPC Server.lvclass">)  [unwired: 7 in]
            n136 = Unbundle By Name(w411) -> ("gRPC Read"=w414:refnum<class "gRPC Read.lvclass">)
            n137 = call "rqp_Start Exiting.vi"("Caller in"=w411, "error in"=w413, "gRPC Read in"=w414) -> ("error out"=w412:errorcluster, "dup Caller out"=w410:refnum<class "gRPC Server.lvclass">)  [unwired: 6 in, 1 out]
          }
        }
        n138 = call-dynamic "Error Handler.vi"("gRPC Server"=w72, "error_in"=w74) -> ("error out"=w77:errorcluster, "Stop Loop"=w70:bool, "gRPC Server out"=w76:refnum<class "gRPC Server.lvclass">)  [unwired: 7 in]
      }
      n139 = call-dynamic "Setup EHL.vi"("Worker"=w27) -> ("Worker out"=w23:refnum<class "gRPC Server.lvclass">)  [unwired: 14 in]
      n140 = while "Event Handling Loop" {
        shift-right: [w36] -> w21
        shift-left: w22 -> [w35]
        tunnel: [w31] -> w20
        tunnel: errorcluster {"status"=FALSE, "code"=0, "source"=""} ("error constant") -> [w33]
        shift-right: [w29] -> _
        shift-left: w23 -> [w34]
        stop <- w28 stop-if-true
        # "Event Handling Loop"
        n141 = event shown="[2] <New Session>: User Event" {
          selector: w35 -> [_ _ w54 _]
          dyn-events: [_ _ w53 _] -> w36
          timeout: _ -> [_ _ _ _]
          tunnel: [w40 w47 w49 w66] -> w32
          tunnel: w33 -> [w41 w46 w51 w67]
          tunnel: w34 -> [w39 w45 w60 w65]
          tunnel: [w38 w44 w60 w64] -> w30
          event User Event {
            # "This case and its contents must always be included in every EHL that you use, so that the framework can automatically stop the EHL."
            # "EHL Stop Event. This EHL exits from this case."
            n142 = event-data() -> ("Stop Event Data"=w37:variant)  [unwired: 1 in]
            n143 = call-dynamic "EHL Stop - EHL Case.vi"("error in"=w41, "Stop Event Data"=w37, "Worker"=w39) -> ("error out"=w40:errorcluster, "Worker out"=w38:refnum<class "gRPC Server.lvclass">)  [unwired: 7 in]
          }
          event Panel Close? {
            # "Use this VI when you want to exit this Worker. This VI will call the Start Exiting case of this Worker. This is the correct way to exit your Worker."
            # "Calls the Start Exiting case of this Worker. This will start the exiting sequence of this Worker."
            n144 = event-data() -> ()  [unwired: 1 in, 1 out]
            n145 = property class="gRPC Server"(reference=w45) -> (reference out=w43:refnum<class "gRPC Server.lvclass">, "Accessors:Read:Public API:Queue"=w42:refnum<class "Message Queue.lvclass">)  [unwired: 1 in, 1 out]
            n146 = call-dynamic "Worker Start Exiting.vi"("error_in"=w46, "Message Queue"=w42, "Worker"=w43) -> ("error out"=w47:errorcluster, "dup Worker out"=w44:refnum<class "gRPC Server.lvclass">)  [unwired: 7 in]
            n147 = event-data("Discard?"=TRUE) -> ()  [unwired: 1 in, 1 out]
          }
          event User Event {
            # "Register gRPC Server to listen for incoming gRPC Client connections"
            n148 = event-data() -> ("gRPC services out"=w56:refnum<class "ServiceBase.lvclass">[])  [unwired: 1 in]
            n149 = Index Array(array=w56) -> (element=w55:refnum<class "ServiceBase.lvclass">)  [unwired: 1 in]
            n150 = To More Specific Class(target class=refnum<class "Session.lvclass"> refnum ("Generated_server.lvlib:Session.lvclass"), reference=w55, error in=w51) -> (specific class reference=w57:refnum<class "Session.lvclass">, error out=w50:errorcluster)
            n151 = call "Read Server RPC Methods.vi"("error in (no error)"=w50, "gRPC service in"=w57) -> ("error out"=w49:errorcluster, "Server RPC Methods"=w59:T51)  [unwired: 7 in, 1 out]
            n152 = Unbundle By Name(w59) -> ("Session Connect gRPC UE"=w52:refnum<user-event>)
            n153 = register-events(reference=w54, w52) -> (reference out=w53:refnum<event-registration>)  [unwired: 3 in, 1 out]
          }
          event User Event {
            # "A gRPC Client has connected to gRPC Server."
            n154 = event-data() -> ("gRPCid"=w61:T2)  [unwired: 1 in]
            n155 = Bundle By Name(cluster=T1 {"gRPC ID"=0} ("Data"), "gRPC ID"=w61) -> (w62:T1)
            n156 = call "rql_New Client Connection.vi"("error in"=w67, "Data in"=w62, "gRPC Server in"=w65) -> ("error out"=w66:errorcluster, "dup gRPC Server out"=w64:refnum<class "gRPC Server.lvclass">)  [unwired: 7 in]
          }
        }
        n157 = call-dynamic "Error Handler.vi"("gRPC Server"=w30, "error_in"=w32) -> ("error out"=w31:errorcluster, "Stop Loop"=w28:bool, "gRPC Server out"=w29:refnum<class "gRPC Server.lvclass">)  [unwired: 7 in]
      }
    }
    frame Error {
      n158 = call-dynamic "Error Handler.vi"("gRPC Server"=w426, "error_in"=w428) -> ("error out"=w427:errorcluster, "gRPC Server out"=w425:refnum<class "gRPC Server.lvclass">)  [unwired: 7 in, 1 out]
    }
  }
  n159 = Unregister For Events(event registration refnum=w11, error in=w10) -> (error out=w9:errorcluster)
  n160 = Merge Errors(w9, w17) -> (w19:errorcluster)
  n161 = call-dynamic "Exited Notify and Cleanup.vi"("error_in"=w19, "Worker"=w18) -> ("error out"=→"error out":errorcluster, "dup Worker out"=→"gRPC Server out":refnum<class "gRPC Server.lvclass">)  [unwired: 8 in]
